vi "Read 1D Barcode.vi"() -> ()   [LabVIEW 2017]
doc: "This example shows how to use the IMAQ Read Barcode VI to locate and read standard 1D barcodes."
uses:
  <vilib>/vision/Instrument.llb/Barcode Search Options.ctl
  <vilib>/vision/NI_Vision_Development_Module.lvlib
panel:
  out "Barcode ANSI/CEN/ISO Grading Report":T1(array[cluster])
  out "Barcode Read":cluster{"Data":string, "Barcode Type":string}[](array[cluster])
  out "Number of Barcodes Found":u32
  out "Image":T2(plugin-control)
  in  "Delay (s.)":dbl(slide)=0.4897959183673469 scale=0.0..2.0
  in  "Stop":bool
  # "Overview: Demonstrate the use of the Read Barcode 2 function of Vision Development Module.\nRequirements: Vision Development Module\nInstructions: Run the VI."
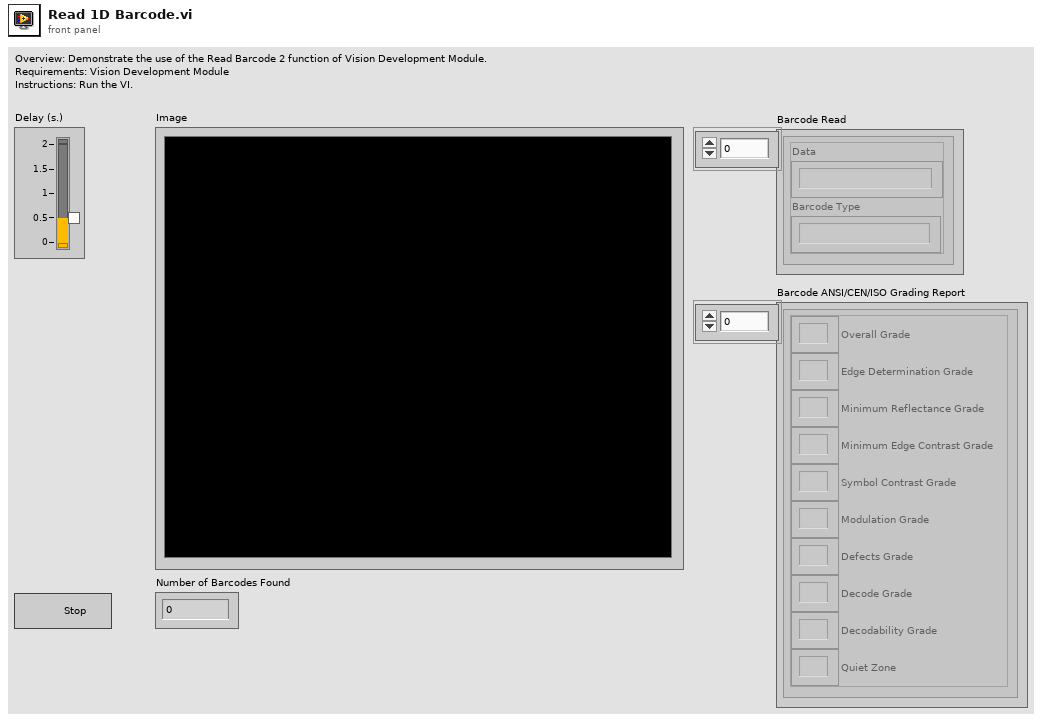
[diagram p1: front panel]
types:
  T1 = cluster{"Overall Grade":string, "Edge Determination Grade":string, "Minimum Reflectance Grade":string, "Minimum Edge Contrast Grade":string, "Symbol Contrast Grade":string, "Modulation Grade":string, "Defects Grade":string, "Decode Grade":string, "Decodability Grade":string, "Quiet Zone":string}[]
  T2 = typedef "IMAQ Image.ctl" = refnum<image>
  T3 = cluster{"Calculate Grading Report":bool, "Scan Width ":i32}
  T4 = typedef "Barcode Search Options.ctl" = cluster{"Min Bar Width":u32, "Min Edge Strength":u32, "Min Bars":u32, "Skip Location Search?":bool}
  T5 = cluster{"Data":string, "Special Char 1":string, "Special Char 2":string, "Checksum(s)":string, "Barcode Type":u32, "Confidence Level":sgl, "Bounding Box":cluster{"x":sgl, "y":sgl}[]}[]
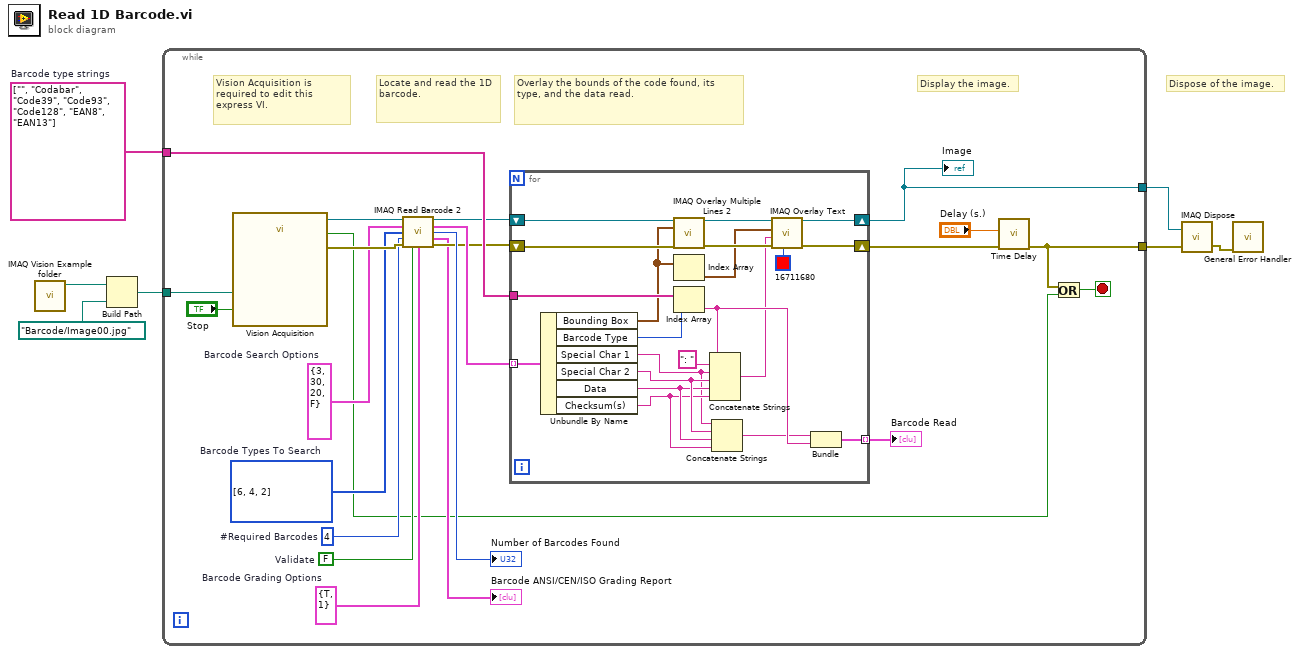
[diagram p0: block diagram]
diagram:
  w3 = string[] ["", "Codabar", "Code39", "Code93", "Code128", "EAN8", "EAN13"]  # Barcode type strings
  # "Dispose of the image."
  n1 = call "IMAQ Vision Example folder.vi"() -> ("Example Image Path"=w7:path)  [unwired: 11 in]
  n2 = Build Path(base path=w7, name or relative path=path "Barcode/Image00.jpg" ("appended path")) -> (appended path=w4:path)
  n3 = while {
    tunnel: [w15] -> w6
    tunnel: [w9] -> w2
    tunnel: w4 -> [w27]
    tunnel: w3 -> [w23]
    stop <- w29 stop-if-true
    w12 = T3 {"Calculate Grading Report"=TRUE, "Scan Width "=1}  # Barcode Grading Options
    w13 = T4 {"Min Bar Width"=3, "Min Edge Strength"=30, "Min Bars"=20, "Skip Location Search?"=FALSE}  # Barcode Search Options
    w25 = u32 4  # #Required Barcodes
    w19 = u32[] [6, 4, 2] items=["Reserved", "Codabar", "Code 39", "Code 93", "Code 128", "EAN 8", "EAN 13", "Interleaved 2 of 5", "MSI", "UPCA", "Pharmacode", "RSS Limited"]  # Barcode Types To Search
    w14 = FALSE  # Validate
    # "Display the image."
    # "Locate and read the 1D barcode."
    # "Vision Acquisition is required to edit this express VI."
    # "Overlay the bounds of the code found, its type, and the data read."
    n4 = call "Vision Acquisition"("Image Path"=w27, "Stop (F)"="Stop") -> ("Image Out"=w21:T2, "Stopped"=w8:bool, "error out"=w26:errorcluster)  [unwired: 23 in]
    n5 = call "IMAQ Read Barcode 2"("Image"=w21, "Barcode Search Options"=w13, "Barcode Types To Search"=w19, "Num of Required Barcodes"=w25, "error in (no error)"=w26, "Validate"=w14, "Barcode Grading Options"=w12) -> ("Image (duplicate)"=w22:T2, "Barcodes"=w24:T5, "Num of Barcodes"=→"Number of Barcodes Found":u32, "Barcode ANSI/CEN/ISO Grading Report"=→"Barcode ANSI/CEN/ISO Grading Report":T1, "error out"=w18:errorcluster)  [unwired: 4 in]
    n6 = for {
      tunnel: w24 -> [w50] mode=indexing
      tunnel: w23 -> [w49]
      shift-right: [w45] -> w15
      shift-left: w22 -> [w41]
      shift-right: [w42] -> w17
      shift-left: w18 -> [w44]
      tunnel: [w37] -> w11 mode=indexing
      n7 = Unbundle By Name(w50) -> ("Bounding Box"=w40:cluster{"x":sgl, "y":sgl}[], "Barcode Type"=w38:u32, "Special Char 1"=w30:string, "Special Char 2"=w34:string, "Data"=w33:string, "Checksum(s)"=w32:string)
      n8 = call "IMAQ Overlay Multiple Lines 2"("Image"=w41, "Line End Points"=w40, "error in (no error)"=w44) -> ("Image Out"=w47:T2, "error out"=w43:errorcluster)  [unwired: 11 in]
      n9 = Index Array(array=w40) -> (element=w39:cluster{"x":sgl, "y":sgl})  [unwired: 1 in]
      n10 = Index Array(array=w49, index=w38) -> (element=w36:string)
      n11 = Concatenate Strings(w36, ": " ("string"), w30, w34, w33, w32) -> (w35:string)
      n12 = Concatenate Strings(w30, w34, w33, w32) -> (w31:string)
      n13 = call "IMAQ Overlay Text"("Text Color (black)"=u32 16711680, "error in (no error)"=w43, "String"=w35, "Origin"=w39, "Image"=w47) -> ("error out"=w42:errorcluster, "Image Out"=w45:T2)  [unwired: 5 in]
      n14 = Bundle(w31, w36) -> (w37:cluster{string, string})  [unwired: 1 in]
    }
    "Image" <- w15
    "Barcode Read" <- w11
    n15 = call "Time Delay"("error in (no error)"=w17, "Delay Time (s)"="Delay (s.)") -> ("error out"=w9:errorcluster)  [unwired: 9 in]
    n16 = Or(x=w9, y=w8) -> (x .or. y?=w29:bool)
  }
  n17 = call "IMAQ Dispose"("Image"=w6, "error in (no error)"=w2) -> ("error out"=w1:errorcluster)  [unwired: 1 in, 3 out]
  n18 = call <vilib>:"General Error Handler.vi"("error in (no error)"=w1) -> ()  [unwired: 10 in, 5 out]
